vi "getNewValueXML.vi"(8 "error in (no error)":errorcluster, 11 "ScriptEvent in":refnum<class "ScriptEvent.lvclass">) -> (0 "error out":errorcluster, 2 "newValueXML":refnum<class "xmlNode.lvclass">, 3 "ScriptEvent out":refnum<class "ScriptEvent.lvclass">)   [LabVIEW 2011, in "Tools.lvlib" / "Scripting.lvlib" / "ScriptEvent.lvclass"]
uses:
  ScriptEvent.lvclass
  xmlNode/xmlNode.lvclass
  ScriptEvent.lvclass/ScriptEvent.ctl
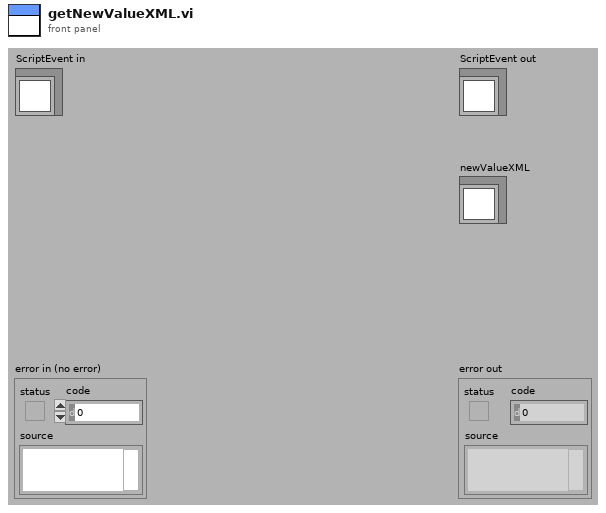
[diagram p1: front panel]
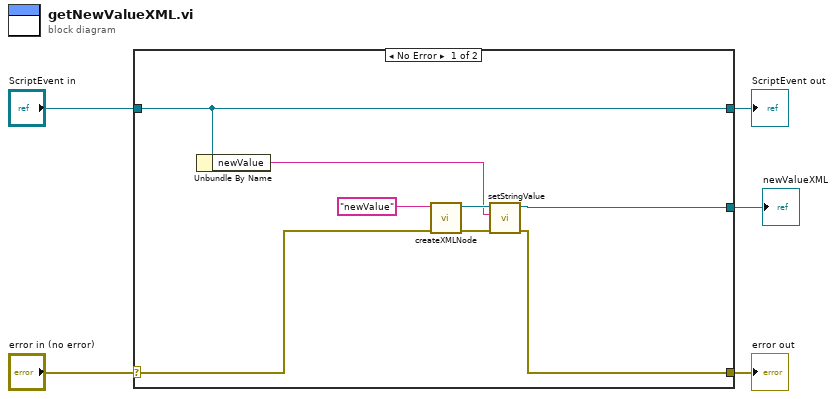
[diagram p0: block diagram]
diagram:
  n1 = case shown="No Error" "error in (no error)" {
    selector: "error in (no error)" -> [w9 w15]
    tunnel: [w8 w15] -> w4
    tunnel: [w7 w14] -> w2
    tunnel: "ScriptEvent in" -> [w7 w14]
    tunnel: [w10 _] -> w1
    frame No Error {
      n2 = Unbundle By Name(w7) -> ("newValue"=w6:string)
      n3 = call "createXMLNode.vi"("error in (no error)"=w9, "name"="newValue") -> ("error out"=w11:errorcluster, "xmlNode out"=w12:refnum<class "xmlNode.lvclass">)  [unwired: 8 in]
      n4 = call-dynamic "setStringValue.vi"("error in (no error)"=w11, "stringValue"=w6, "xmlNode.lvclass in"=w12) -> ("error out"=w8:errorcluster, "xmlNode.lvclass out"=w10:refnum<class "xmlNode.lvclass">)  [unwired: 7 in]
    }
    frame Error {
    }
  }
  "error out" <- w4
  "ScriptEvent out" <- w2
  "newValueXML" <- w1
